vi "(SubVI) Pre-Add Data For Fixed-Window Filters_YCC.vi"(4 "All add in the tail?":bool, 5 "Avg points":i32, 7 "Signal":dbl[](array[numeric])) -> (1 "loop # for Silding window":dbl, 3 "added-Signal":dbl[](array[numeric]))   [LabVIEW 2014]
panel:
  out "# of terms to be added into head":i32
  out "# of terms to be added into tail":i32
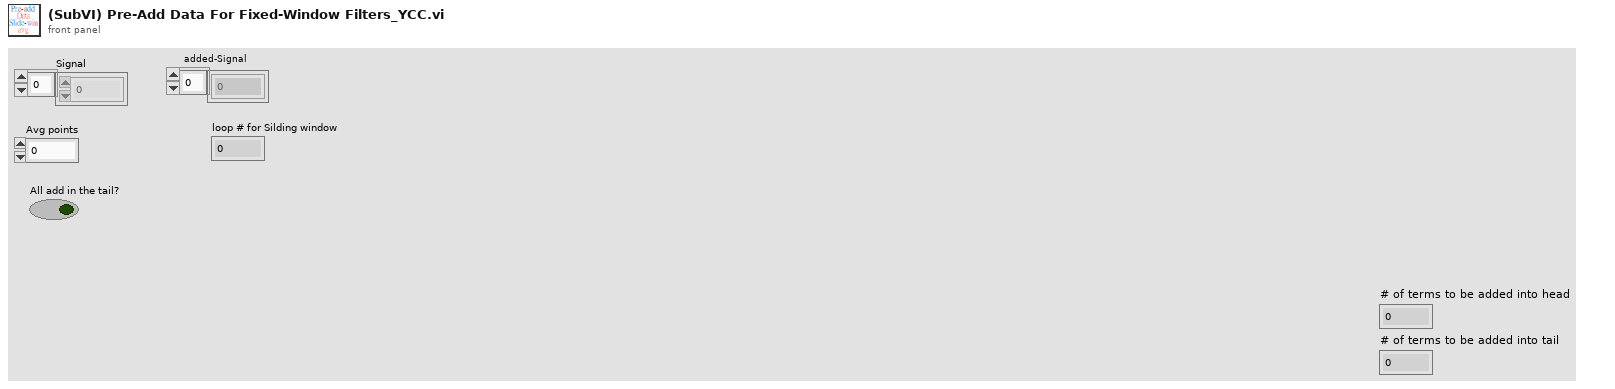
[diagram p1: front panel]
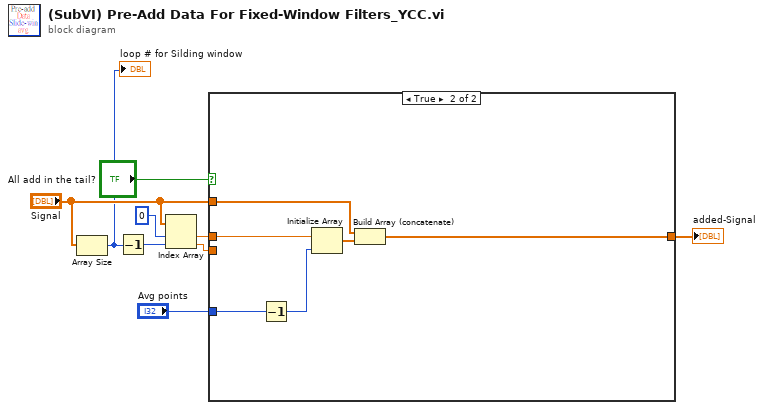
[diagram p0: block diagram]
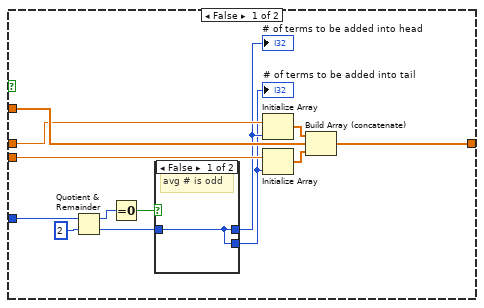
[diagram p2: hidden frame]
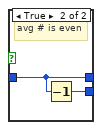
[diagram p3: hidden frame]
diagram:
  n1 = Array Size(array="Signal") -> (size(s)=w2:i32)
  "loop # for Silding window" <- w2
  n2 = Decrement(x=w2) -> (x-1=w7:i32)
  n3 = Index Array(array="Signal", index #1=0 ("index"), index #2=w7) -> (element #1=w4:dbl, element #2=w5:dbl)
  n4 = case shown="True" "All add in the tail?" {
    tunnel: [w22 w26] -> w9
    tunnel: "Signal" -> [w21 w27]
    tunnel: w5 -> [w18 _]
    tunnel: w4 -> [w17 w31]
    tunnel: "Avg points" -> [w16 w30]
    frame False {
      n5 = Quotient & Remainder(x=w16, y=2) -> (x-y*floor(x/y)=w14:i32, floor(x/y)=w15:i32)
      n6 = Equal To 0?(x=w14) -> (x = 0?=w13:bool)
      n7 = case shown="False" w13 {
        tunnel: [w23 w25] -> w11
        tunnel: w15 -> [w23 w25]
        tunnel: [w23 w24] -> w10
        frame False {
          # "avg # is odd"
        }
        frame True {
          # "avg # is even"
          n8 = Decrement(x=w25) -> (x-1=w24:i32)
        }
      }
      "# of terms to be added into head" <- w11
      "# of terms to be added into tail" <- w10
      n9 = Initialize Array(w17, w11) -> (w19:dbl[])
      n10 = Initialize Array(w18, w10) -> (w20:dbl[])
      n11 = Build Array (concatenate)(w19, w21, w20) -> (w22:dbl[])
    }
    frame True {
      n12 = Decrement(x=w30) -> (x-1=w29:i32)
      n13 = Initialize Array(w31, w29) -> (w28:dbl[])
      n14 = Build Array (concatenate)(w27, w28) -> (w26:dbl[])
    }
  }
  "added-Signal" <- w9
